vi "PCert-ConfigPageNF-Launch.vi"(6 "ERP-Container-UI in":refnum<class "PCert-Container-UI.lvclass">, 7 "Actor Name":string, 8 "error in (no error)":errorcluster, 9 "Container Address":string, 10 "Database Address":string, 11 "Configuration Page VI Filepath":path) -> (0 "error out":errorcluster, 2 "PageID":string, 4 "ERP-Container-UI out":refnum<class "PCert-Container-UI.lvclass">)   [LabVIEW 2013, in "PCert-ConfigPageNF.lvclass"]
uses:
  PCert-ConfigPageNF.lvclass
  PCert-Container-UI.lvclass
  ftw-dataflow/Actor/src/Connector/FTW-ActorConnector.lvclass
panel:
  in  "Configuration":string="{\n  \"Identity\": \"ActorName\",\n  \"InboxAddress\": \"tcp://127.0.0.1:*\",\n  \"PublisherAddress\": \"tcp://127.0.0.1:*\",\n  \"DebugEnableInboxLogging\": false,\n  \"DebugEnableJobLogging\": false,\n  \"DebugShowPanel\": false\n}"
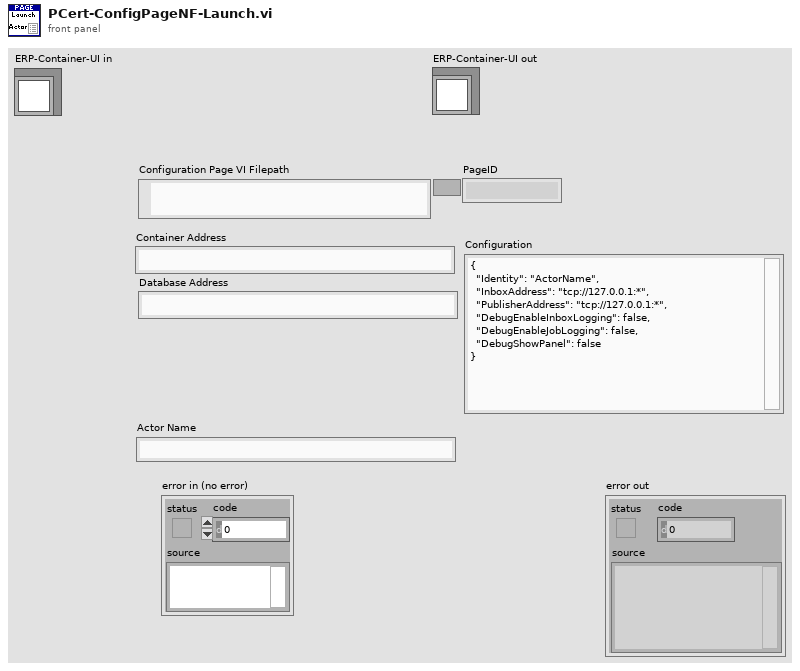
[diagram p1: front panel]
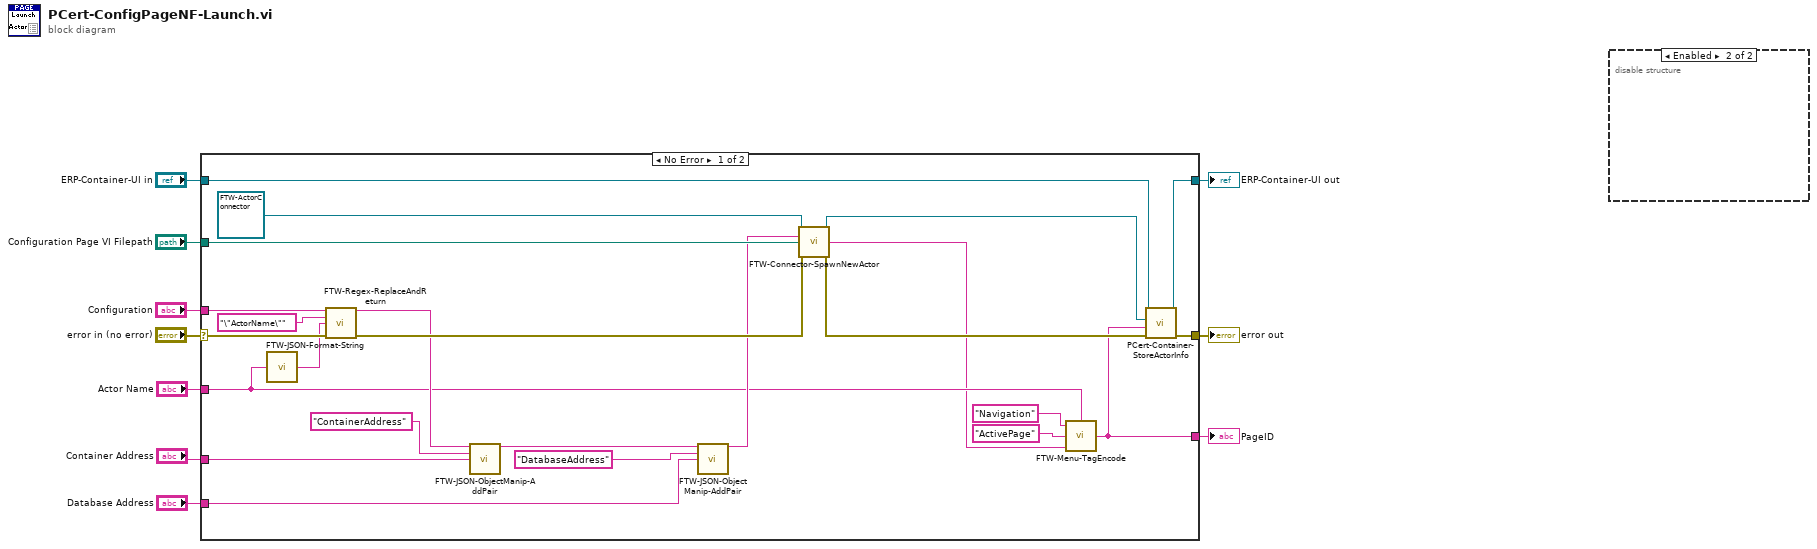
[diagram p0: block diagram]
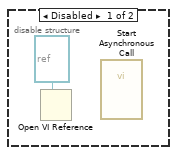
[diagram p2: hidden frame]
diagram:
  n1 = case shown="No Error" "error in (no error)" {
    selector: "error in (no error)" -> [w23 w35]
    tunnel: [w27 w35] -> w9
    tunnel: "Configuration" -> [w24 _]
    tunnel: "Container Address" -> [w33 _]
    tunnel: "Configuration Page VI Filepath" -> [w30 _]
    tunnel: [w20 _] -> w6
    tunnel: "ERP-Container-UI in" -> [w26 _]
    tunnel: [w25 _] -> w4
    tunnel: "Actor Name" -> [w14 _]
    tunnel: "Database Address" -> [w17 _]
    frame No Error {
      n2 = call "FTW-JSON-Format-String.vi"("LabVIEW String"=w14) -> ("JSON String"=w13:string)
      n3 = call "FTW-Regex-ReplaceAndReturn.vi"("String"=w24, "Search for (Regular Expression)"="\"ActorName\"", "Replace with"=w13, "error in"=w23) -> ("String out"=w21:string, "error out"=w22:errorcluster)  [unwired: 7 in, 3 out]
      n4 = call "FTW-JSON-ObjectManip-AddPair.vi"("Input JSON Object"=w21, "Key"="ContainerAddress", "Value"=w33) -> ("Output JSON Object"=w19:string)  [unwired: 11 in, 1 out]
      n5 = call "FTW-JSON-ObjectManip-AddPair.vi"("Input JSON Object"=w19, "Key"="DatabaseAddress", "Value"=w17) -> ("Output JSON Object"=w16:string)  [unwired: 11 in, 1 out]
      n6 = call "FTW-Connector-SpawnNewActor.vi"("FTW Actor Connector Type"=refnum<class "FTW-ActorConnector.lvclass"> refnum ("Featherweight Actor:FTW Actor Connector"), "Configuration"=w16, "Actor VI Filepath"=w30, "error in"=w22) -> ("FTW Actor Connector"=w11:refnum<class "FTW-ActorConnector.lvclass">, "Instance Inbox Address"=w12:string, "error out"=w28:errorcluster)  [unwired: 7 in, 2 out]
      n7 = call "FTW-Menu-TagEncode.vi"("Actor Name"=w14, "Payload"=w12, "Command"="ActivePage", "Class"="Navigation") -> ("Tag"=w20:string)
      n8 = call "PCert-Container-StoreActorInfo.vi"("error in (no error)"=w28, "ActorID"=w20, "FTW Actor Connector"=w11, "ERP-Container-UI in"=w26) -> ("error out"=w27:errorcluster, "ERP-Container-UI out"=w25:refnum<class "PCert-Container-UI.lvclass">)  [unwired: 6 in]
    }
    frame Error {
    }
  }
  "error out" <- w9
  "PageID" <- w6
  "ERP-Container-UI out" <- w4
  n9 = disable-structure shown="Enabled" {
    frame Disabled {
      n10 = Open VI Reference(type specifier VI Refnum (for type only)=refnum<vi> refnum) -> ()  [unwired: 5 in, 2 out]
      n11 = call-by-ref "Start Asynchronous Call"() -> ()  [unwired: 17 in, 3 out]
    }
    frame Enabled {
    }
  }
